vi "NNF_Draw_Rectangle.vi"(5 "font_size":sgl=20.0, 6 "Labels":string[](array[string])=["aeroplane", "bicycle", "bird", "boat", "bottle", "bus", "car", "cat", "chair", "cow", "diningtable", "dog", "horse", "motorbike", "person", "pottedplant", "sheep", "sofa", "train", "tvmonitor"], 7 "Border_Width":u32=4, 8 "error in (no error)":errorcluster, 10 "Draw_Boxes":T1[](array[typedef]) {"BBox"."x" format="%#_4p"; "BBox"."y" format="%#_4p"; "BBox"."w" format="%#_4p"; "BBox"."h" format="%#_4p"}, 11 "Img in":T3=refnum) -> (0 "error out":errorcluster, 3 "Img out":T3)   [LabVIEW 2020]
doc: "Draws bounding box regtangles around objects on the image based on BBox input information ."
uses:
  <vilib>/vision/Image Controls.llb/IMAQ Image.ctl
  <vilib>/Ngene/Deep Learning Toolkit/Toolkit/NN_Data/API/Data/Detection_Types/NN_BBox_Detection.ctl
  <vilib>/Ngene/Deep Learning Toolkit/Toolkit/NN_Data/API/Data/Detection_Types/NN_BBox.ctl
  <vilib>/Ngene/Deep Learning Toolkit/Toolkit/NN_Data/API/NN_Dims(C,H,W).ctl
  <vilib>/Ngene/Deep Learning Toolkit/Toolkit/Deep_Learning_Toolkit_by_Ngene.lvlib
panel:
  out "Exec_Time(s)":dbl=0.000148600014654221
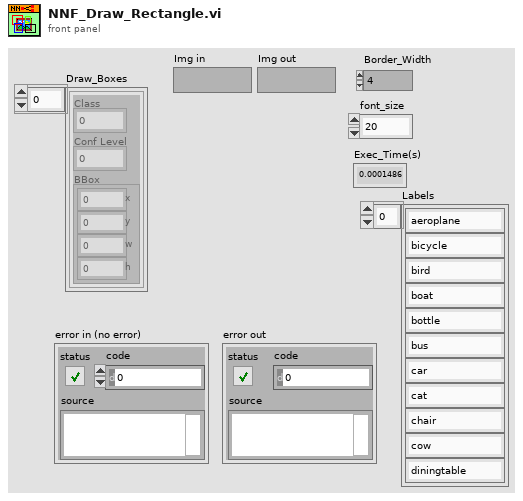
[diagram p1: front panel]
types:
  T1 = typedef "Deep_Learning_Toolkit_by_Ngene.lvlib/NN_BBox_Detection.ctl" = cluster{"Class":i32, "Conf Level":sgl, "BBox":T2}
  T2 = typedef "Deep_Learning_Toolkit_by_Ngene.lvlib/NN_BBox.ctl" = cluster{"x":sgl, "y":sgl, "w":sgl, "h":sgl}
  T3 = typedef "IMAQ Image.ctl" = refnum<image>
  T4 = typedef "Deep_Learning_Toolkit_by_Ngene.lvlib/NN_Dims(C,H,W).ctl" = cluster{"C":i32, "H":i32, "W":i32}
  T5 = cluster{"Desired Font (Application)":enum16{"User-specified Font", "Application Font", "System Font", "Dialog Font"}, "[User-specified Font]":cluster{"Font Name":string, "Size":i16, "Strikeout?":bool, "Italic?":bool, "Underline?":bool, "Outline?":bool, "Shadow?":bool, "Bold?":bool, "Rotation Angle":dbl}, "Horizontal Alignment":i16, "Vertical Alignment":i16}
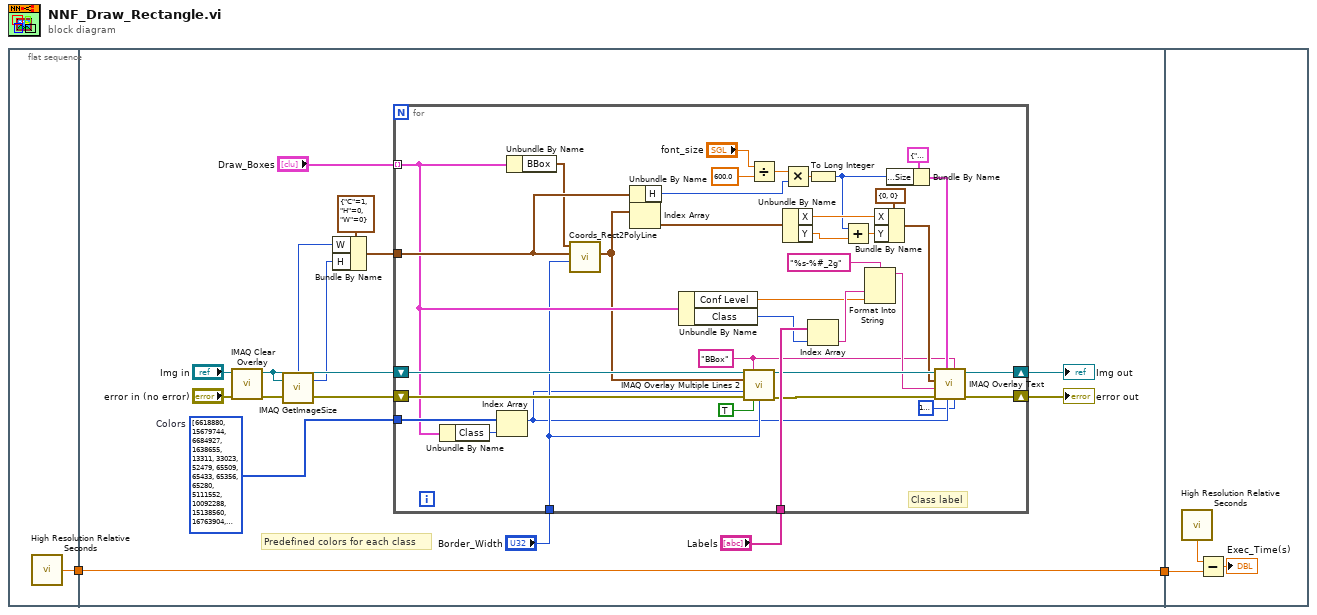
[diagram p0: block diagram]
diagram:
  n1 = flat-sequence {
    tunnel: [w3] -> w2
    tunnel: w2 -> [w7]
    tunnel: [w7] -> w1
    tunnel: w1 -> [w58]
    frame #0 {
      n2 = call <vilib>:"High Resolution Relative Seconds.vi"() -> ("relative seconds"=w3:dbl)
    }
    frame #1 {
      w14 = u32[] [6618880, 15679744, 6684927, 1638655, 13311, 33023, 52479, 65509, 65433, 65356, 65280, 5111552, 10092288, 15138560, 16763904, 16744192, 16724736, 16711680, 16711680, 16711680]  # Colors
      # "Predefined colors for each class"
      n3 = call "IMAQ Clear Overlay"("Image"="Img in") -> ("Image Out"=w10:T3)  [unwired: 9 in, 1 out]
      n4 = call "IMAQ GetImageSize"("Image"=w10, "error in (no error)"="error in (no error)") -> ("Y Resolution"=w8:i32, "X Resolution"=w9:i32, "error out"=w11:errorcluster)  [unwired: 2 in]
      n5 = Bundle By Name(cluster=T4 {"C"=1, "H"=0, "W"=0} ("In_Dims"), "W"=w9, "H"=w8) -> (w13:T4)
      n6 = for {
        tunnel: w14 -> [w55]
        shift-right: [w54] -> w18
        shift-left: w11 -> [w51]
        shift-right: [w53] -> w17
        shift-left: w10 -> [w50]
        tunnel: w13 -> [w52]
        tunnel: "Draw_Boxes" -> [w49] mode=indexing
        tunnel: "Border_Width" -> [w47]
        tunnel: "Labels" -> [w46]
        w31 = "BBox" ("Group")
        # "Class label"
        n7 = Unbundle By Name(w49) -> ("Class"=w48:i32)
        n8 = Index Array(array=w55, index=w48) -> (element=w20:u32)
        n9 = Unbundle By Name(w49) -> ("BBox"=w32:T2)
        n10 = call <vilib>:"Coords_Rect2PolyLine.vi"("Border_Width"=w47, "In_Dims"=w52, "BBox"=w32) -> ("PolyLine"=w25:cluster{"X":dbl, "Y":dbl}[])  [unwired: 8 in]
        n11 = Unbundle By Name(w52) -> ("H"=w26:i32)
        n12 = Index Array(array=w25) -> (element=w24:cluster{"X":dbl, "Y":dbl})  [unwired: 1 in]
        n13 = Unbundle By Name(w49) -> ("Conf Level"=w21:sgl, "Class"=w23:i32)
        n14 = call "IMAQ Overlay Multiple Lines 2"("Image"=w50, "Group"=w31, "Line End Points"=w25, "Color"=w20, "error in (no error)"=w51, "Maintain Width?"=TRUE, "Width"=w47) -> ("Image Out"=w45:T3, "error out"=w44:errorcluster)  [unwired: 7 in]
        n15 = Divide(x="font_size", y=sgl 600.0) -> (x/y=w34:sgl)
        n16 = Multiply(x=w34, y=w26) -> (x*y=w35:sgl)
        n17 = Unbundle By Name(w24) -> ("X"=w29:dbl, "Y"=w28:dbl)
        n18 = To Long Integer(number=w35) -> (32bit integer=w27:i32)
        n19 = Index Array(array=w46, index=w23) -> (element=w22:string)
        n20 = Add(x=w27, y=w28) -> (x+y=w41:dbl)
        n21 = Format Into String(format string="%s-%#_2g", w22, w21) -> (resulting string=w39:string)  [unwired: 2 in, 1 out]
        n22 = Bundle By Name(cluster=cluster{"X":i32, "Y":i32} {"X"=0, "Y"=0} ("Origin"), "X"=w29, "Y"=w41) -> (w42:cluster{"X":i32, "Y":i32})
        n23 = Bundle By Name(cluster=T5 {"Desired Font (Application)"=enum."User-specified Font", "[User-specified Font]"={"Font Name"="", "Size"=18, "Strikeout?"=FALSE, "Italic?"=FALSE, "Underline?"=FALSE, "Outline?"=FALSE, "Shadow?"=FALSE, "Bold?"=TRUE, "Rotation Angle"=0.0}, "Horizontal Alignment"=0, "Vertical Alignment"=0} ("Font, Size & Style"), "[User-specified Font].Size"=w27) -> (w37:T5)
        n24 = call "IMAQ Overlay Text"("BG Color (Transparent)"=u32 16777216, "Group"=w31, "Text Color (black)"=w20, "Font, Size & Style"=w37, "error in (no error)"=w44, "String"=w39, "Origin"=w42, "Image"=w45) -> ("error out"=w54:errorcluster, "Image Out"=w53:T3)  [unwired: 2 in]
      }
      "error out" <- w18
      "Img out" <- w17
    }
    frame #2 {
      n25 = call <vilib>:"High Resolution Relative Seconds.vi"() -> ("relative seconds"=w57:dbl)
      n26 = Subtract(x=w57, y=w58) -> (x-y=→"Exec_Time(s)":dbl)
    }
  }
